vi "Rename- failureDBs files.vi"() -> (3 "Path to copy to!":path)   [LabVIEW 2012]
uses:
  <vilib>/regexp/Match Regular Expression.xnode
panel:
  out "concatenated string":string
  in  "Desired location?":string="E:\\UGDGNEW\\NATIVE2013--IAT_Windows_7_32.xml"
  in  "Full p4v path":string="//labview/branches/2013/dev/tests/auto/Testsuite/Report/IAT_Windows_7_32.xml "
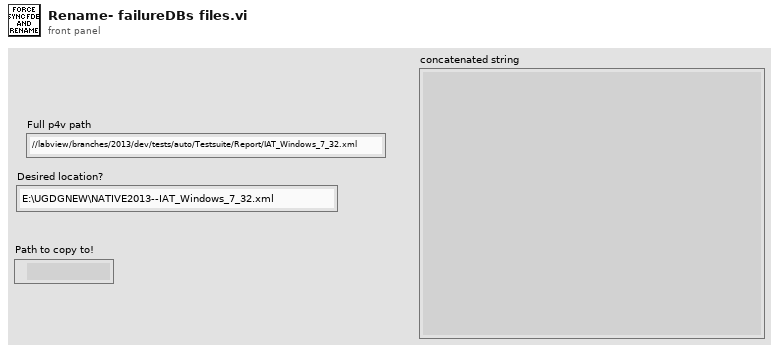
[diagram p1: front panel]
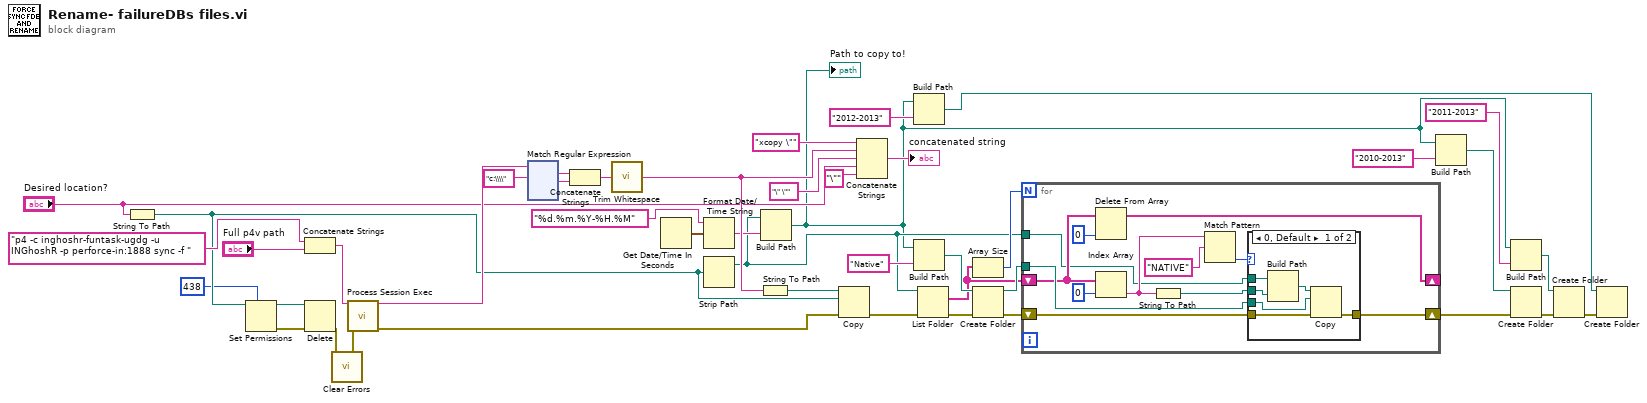
[diagram p0: block diagram]
diagram:
  n1 = String To Path(string="Desired location?") -> (path=w5:path)
  n2 = Set Permissions(7:i16 438 ("permissions"), 11:w5) -> (0:w3:errorcluster, 3:w2:path)  [unwired: 3 in]
  n3 = Concatenate Strings("p4 -c inghoshr-funtask-ugdg -u INGhoshR -p perforce-in:1888 sync -f ", "Full p4v path") -> (w40:string)
  n4 = Delete(path (use dialog)=w2, error in=w3) -> (error out=w6:errorcluster)  [unwired: 3 in, 2 out]
  n5 = call <vilib>:"Clear Errors.vi"("error in (no error)"=w6) -> ("error out"=w1:errorcluster)  [unwired: 6 in]
  n6 = call "Process Session Exec.vi"("command line"=w40, "error in (no error)"=w1) -> ("stdout"=w43:string, "error out"=w44:errorcluster)  [unwired: 9 in, 3 out]
  n7 = xnode "Match Regular Expression"("input string"=w43, "regular expression"="c:\\\\") -> ("whole match"=w25:string, "after match"=w24:string)  [unwired: 4 in, 3 out]
  n8 = Concatenate Strings(w25, w24) -> (w35:string)
  n9 = call <vilib>:"Trim Whitespace.vi"("string"=w35) -> ("trimmed string"=w32:string)  [unwired: 1 in]
  n10 = Get Date/Time In Seconds() -> (seconds since 1Jan1904=w11:timestamp)
  n11 = Format Date/Time String(time format string (%c)="%d.%m.%Y-%H.%M", seconds (now)=w11) -> (date/time string=w9:string)  [unwired: 1 in]
  n12 = Strip Path(path=w5) -> (stripped path=w8:path)  [unwired: 1 out]
  n13 = String To Path(string=w32) -> (path=w31:path)
  n14 = Build Path(base path=w8, name or relative path=w9) -> (appended path=w7:path)
  "Path to copy to!" <- w7
  n15 = Copy(8:w44, 10:w5, 11:w31) -> (0:w27:errorcluster)  [unwired: 2 in, 2 out]
  n16 = Concatenate Strings("xcopy \"" ("string"), w32, "\" \"" ("string"), "Desired location?", "\"" ("string")) -> (→"concatenated string":string)
  n17 = Build Path(base path=w7, name or relative path="2012-2013") -> (appended path=w14:path)
  n18 = Build Path(base path=w7, name or relative path="Native") -> (appended path=w33:path)
  n19 = List Folder(path=w8, error in=w27) -> (filenames=w22:string[], error out=w26:errorcluster)  [unwired: 2 in, 2 out]
  n20 = Array Size(array=w22) -> (size(s)=w29:i32)
  n21 = Create Folder(path (use dialog)=w33, error in=w26) -> (created path=w30:path, error out=w28:errorcluster)  [unwired: 1 in, 1 out]
  n22 = for {
    N: w29 -> [_]
    shift-right: [w51] -> _
    shift-left: w22 -> [w53]
    tunnel: w30 -> [w54]
    shift-right: [w50] -> w12
    shift-left: w28 -> [w49]
    tunnel: w8 -> [w46]
    n23 = Delete From Array(array=w53, index=0) -> (array with subset deleted=w51:string[])  [unwired: 1 in, 1 out]
    n24 = Index Array(array=w53, index=0) -> (element=w47:string)
    n25 = String To Path(string=w47) -> (path=w48:path)
    n26 = Match Pattern(string=w47, regular expression="NATIVE") -> (offset past match=w55:i32)  [unwired: 1 in, 3 out]
    n27 = case shown="0, Default" w55 {
      tunnel: w54 -> [w62 _]
      tunnel: w48 -> [w59 _]
      tunnel: w49 -> [w61 w63]
      tunnel: [w60 w63] -> w50
      tunnel: w46 -> [w58 _]
      frame 0, Default {
        n28 = Build Path(base path=w58, name or relative path=w59) -> (appended path=w57:path)
        n29 = Copy(8:w61, 10:w62, 11:w57) -> (0:w60:errorcluster)  [unwired: 2 in, 2 out]
      }
      frame -1 {
      }
    }
  }
  n30 = Build Path(base path=w7, name or relative path="2010-2013") -> (appended path=w19:path)
  n31 = Build Path(base path=w7, name or relative path="2011-2013") -> (appended path=w16:path)
  n32 = Create Folder(path (use dialog)=w19, error in=w12) -> (error out=w21:errorcluster)  [unwired: 1 in, 2 out]
  n33 = Create Folder(path (use dialog)=w16, error in=w21) -> (error out=w15:errorcluster)  [unwired: 1 in, 2 out]
  n34 = Create Folder(path (use dialog)=w14, error in=w15) -> ()  [unwired: 1 in, 3 out]
